vi "LVLibNameFromFilePath.vi"(8 "error in (no error)":errorcluster, 11 "LV File Path":path) -> (0 "error out":errorcluster, 3 "Library Name":string)   [LabVIEW 2023, in "CICD.lvlib"]
uses:
  CICD.lvlib
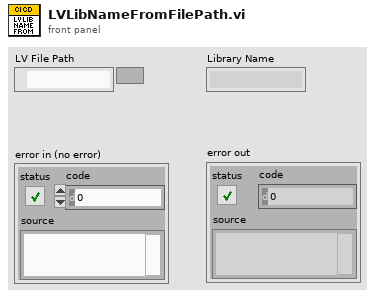
[diagram p1: front panel]
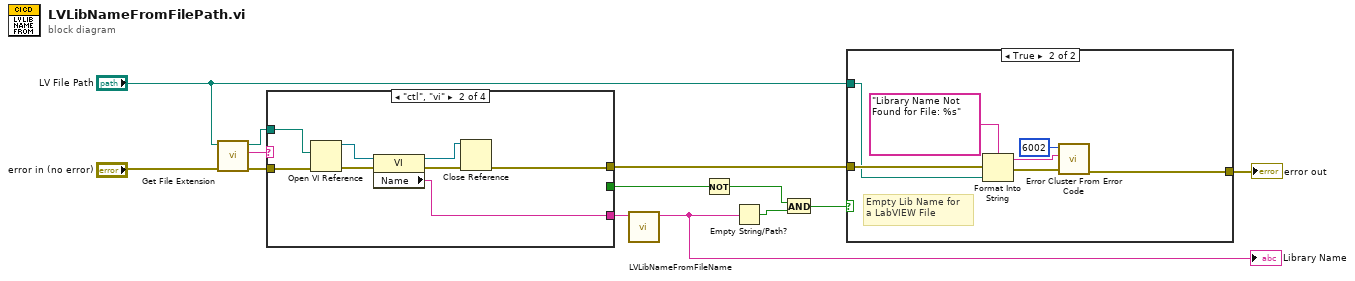
[diagram p0: block diagram]
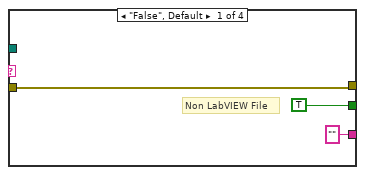
[diagram p3: hidden frame]
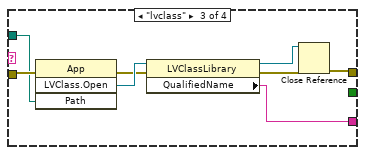
[diagram p4: hidden frame]
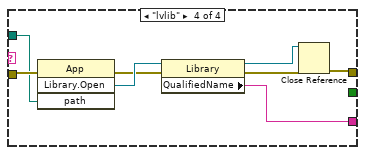
[diagram p5: hidden frame]
diagram:
  n1 = call <vilib>:"Get File Extension.vi"("error in (no error)"="error in (no error)", "file"="LV File Path") -> ("error out"=w12:errorcluster, "lowercase file extension"=w10:string, "dup file"=w11:path)  [unwired: 5 in, 2 out]
  n2 = case shown="\"ctl\", \"vi\"" w10 {
    tunnel: w11 -> [_ w23 w30 w38]
    tunnel: w12 -> [w16 w24 w31 w39]
    tunnel: [w16 w17 w26 w34] -> w7
    tunnel: ["" ("QualifiedName") w20 w28 w36] -> w13
    tunnel: [TRUE _ _ _] -> w4
    frame "False", Default {
      # "Non LabVIEW File"
    }
    frame "ctl", "vi" {
      n3 = Open VI Reference(vi path=w23, error in (no error)=w24) -> (vi reference=w21:refnum<vi>, error out=w22:errorcluster)  [unwired: 4 in]
      n4 = property class="VI"(reference=w21, error in=w22) -> (reference out=w18:refnum<vi>, error out=w19:errorcluster, "Name"=w20:string)
      n5 = Close Reference(reference=w18, error in (no error)=w19) -> (error out=w17:errorcluster)
    }
    frame "lvclass" {
      n6 = invoke class="App" method="LVClass.Open"(error in=w31, "Path"=w30) -> (error out=w29:errorcluster, "LVClass.Open"=w32:refnum<vi>)  [unwired: 2 in, 2 out]
      n7 = property class="LVClassLibrary"(reference=w32, error in=w29) -> (reference out=w25:refnum<vi>, error out=w27:errorcluster, "QualifiedName"=w28:string)
      n8 = Close Reference(reference=w25, error in (no error)=w27) -> (error out=w26:errorcluster)
    }
    frame "lvlib" {
      n9 = invoke class="App" method="Library.Open"(error in=w39, "path"=w38) -> (error out=w37:errorcluster, "Open Library"=w40:refnum<vi>)  [unwired: 2 in, 2 out]
      n10 = property class="Library"(reference=w40, error in=w37) -> (reference out=w33:refnum<vi>, error out=w35:errorcluster, "QualifiedName"=w36:string)
      n11 = Close Reference(reference=w33, error in (no error)=w35) -> (error out=w34:errorcluster)
    }
  }
  n12 = call "LVLibNameFromFileName.vi"("VI Name / CTL Name / LVCLASS Name"=w13) -> ("Library Name"=w8:string)  [unwired: 10 in]
  "Library Name" <- w8
  n13 = Not(x=w4) -> (.not. x?=w2:bool)
  n14 = Empty String/Path?(string/path=w8) -> (empty?=w3:bool)
  n15 = And(x=w2, y=w3) -> (x .and. y?=w1:bool)
  n16 = case shown="True" w1 {
    tunnel: w7 -> [w41 w48]
    tunnel: "LV File Path" -> [_ w44]
    tunnel: [w41 w42] -> w5
    frame False {
    }
    frame True {
      # "Empty Lib Name for\na LabVIEW File"
      n17 = Format Into String(format string="Library Name Not Found for File: %s", error in=w48, w44) -> (resulting string=w43:string, error out=w47:errorcluster)  [unwired: 1 in]
      n18 = call <vilib>:"Error Cluster From Error Code.vi"("error in (no error)"=w47, "error message (\"\")"=w43, "error code (0)"=6002) -> ("error out"=w42:errorcluster)  [unwired: 6 in]
    }
  }
  "error out" <- w5
